vi "Extract Coefs for Network.vi"(9 "Min Array":dbl[](array[numeric]), 11 "Max Array":dbl[](array[numeric])) -> (1 "Y Scaling Vector":dbl[](array[numeric]), 3 "X Scaling Vector":dbl[](array[numeric]))   [LabVIEW 2015, in "Teaching File.lvlib"]
doc: "Extract the scaling information, used to scale inputs and outputs of the network into range 0.2 - 0.8 in which the unipolar sigmoidal activation of neural layers works best."
uses:
  Teaching File/Teaching File.lvlib
  Neural Network.lvclass
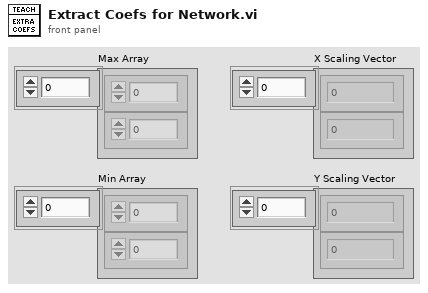
[diagram p1: front panel]
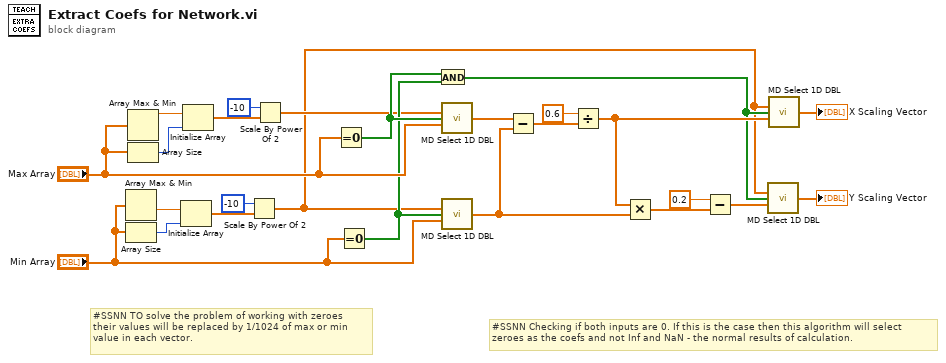
[diagram p0: block diagram]
diagram:
  # "#SSNN TO solve the problem of working with zeroes\ntheir values will be replaced by 1/1024 of max or min\nvalue in each vector."
  # "#SSNN Checking if both inputs are 0. If this is the case then this algorithm will select\nzeroes as the coefs and not Inf and NaN - the normal results of calculation."
  n1 = Array Max & Min(array="Min Array") -> (min value=w21:dbl)  [unwired: 3 out]
  n2 = Array Size(array="Min Array") -> (size(s)=w20:i32)
  n3 = Array Max & Min(array="Max Array") -> (max value=w3:dbl)  [unwired: 3 out]
  n4 = Array Size(array="Max Array") -> (size(s)=w18:i32)
  n5 = Initialize Array(w21, w20) -> (w15:dbl[])
  n6 = Initialize Array(w3, w18) -> (w13:dbl[])
  n7 = Scale By Power Of 2(n=i16 -10, x=w15) -> (x*2^n=w1:dbl[])
  n8 = Scale By Power Of 2(n=i16 -10, x=w13) -> (x*2^n=w5:dbl[])
  n9 = Equal To 0?(x="Max Array") -> (x = 0?=w11:bool[])
  n10 = Equal To 0?(x="Min Array") -> (x = 0?=w10:bool[])
  n11 = And(x=w11, y=w10) -> (x .and. y?=w7:bool[])
  n12 = call "MD Select 1D DBL.vi"("First Array"=w5, "Condition"=w11, "Second Array"="Max Array") -> ("Resulting Array"=w17:dbl[])  [unwired: 12 in]
  n13 = call "MD Select 1D DBL.vi"("First Array"=w1, "Condition"=w10, "Second Array"="Min Array") -> ("Resulting Array"=w2:dbl[])  [unwired: 12 in]
  n14 = Subtract(x=w17, y=w2) -> (x-y=w24:dbl[])
  n15 = Divide(x=0.6, y=w24) -> (x/y=w9:dbl[])
  n16 = Multiply(x=w9, y=w2) -> (x*y=w22:dbl[])
  n17 = Subtract(x=0.2, y=w22) -> (x-y=w6:dbl[])
  n18 = call "MD Select 1D DBL.vi"("First Array"=w1, "Condition"=w7, "Second Array"=w6) -> ("Resulting Array"=→"Y Scaling Vector":dbl[])  [unwired: 12 in]
  n19 = call "MD Select 1D DBL.vi"("First Array"=w1, "Condition"=w7, "Second Array"=w9) -> ("Resulting Array"=→"X Scaling Vector":dbl[])  [unwired: 12 in]
